vi "WaitForInputData.vi"(0 "Input data timeout":i32=-1 caption="Input data timeout (-1) [ms]" min=-1, 11 "Error in":errorcluster caption="Error in (no error)") -> (4 "Input data timed out?":bool, 6 "Input data names":string[](array[string]), 8 "Input data values":variant[](array[variant]), 15 "Error out":errorcluster)   [LabVIEW 2017, in "VILauncher.lvlib"]
doc: "Waits for <B>Input data names</B> and <B>Input data values</B> sent by a launcher to a dynamic VI using the Run or OpenAndRun function.\n\nThe optional <B>Input data timeout</B> specifies how long time to wait for the input data. Set this to -1 (default) to wait indefinitely. If timeout does occur, <B>Input data timed out?</B> will be True.\n\nThis function does not have to be located in the Top-Level dynamic VI, but can be embedded anywhere in the dynamic VI hierarchy. Just be sure to read the input data before timeout of the Run/OpenAndRun function occurs, or else the input data will be lost.\n\nThis VI is reentrant, and it doesn't run if there is an error on <B>Error in</B>.\n\nSteen Schmidt\nGPower\n30/12 2012"
uses:
  VILauncher.lvlib
panel:
  # "Copyright © 2013\nGPower\nSee enclosed license file for terms and conditions"
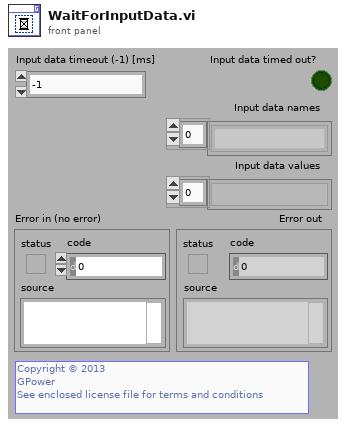
[diagram p1: front panel]
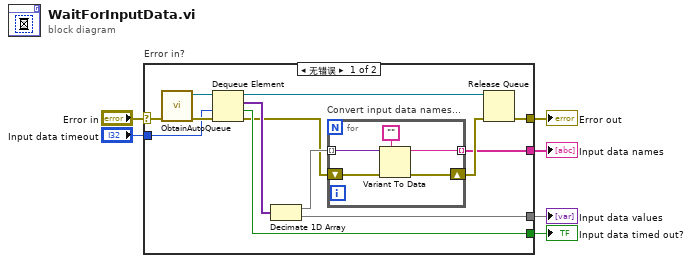
[diagram p0: block diagram]
diagram:
  n1 = case "Error in?" shown="无错误" "Error in" {
    selector: "Error in" -> [w12 w25]
    tunnel: [w16 w25] -> w5
    tunnel: "Input data timeout" -> [w15 _]
    tunnel: [w13 _] -> w3
    tunnel: [w10 _] -> w2
    tunnel: [w7 _] -> w1
    frame No Error {
      n2 = call "ObtainAutoQueue.vi"("Error in"=w12) -> ("Queue"=w18:refnum<queue>, "Error out"=w19:errorcluster)  [unwired: 13 in]
      n3 = Dequeue Element(queue=w18, timeout in ms (-1)=w15, error in (no error)=w19) -> (queue out=w17:refnum<queue>, element=w14:variant[], timed out?=w13:bool, error out=w9:errorcluster)
      n4 = Decimate 1D Array(w14) -> (w11:variant[], w10:variant[])
      n5 = for "Convert input data names..." {
        tunnel: w11 -> [w24] mode=indexing
        shift-right: [w21] -> w8
        shift-left: w9 -> [w22]
        tunnel: [w20] -> w7 mode=indexing
        n6 = Variant To Data(error in=w22, type="", Variant=w24) -> (data=w20:string, error out=w21:errorcluster)
      }
      n7 = Release Queue(queue=w17, error in (no error)=w8) -> (error out=w16:errorcluster)  [unwired: 1 in, 2 out]
    }
    frame Error {
    }
  }
  "Error out" <- w5
  "Input data values" <- w2
  "Input data names" <- w1
  "Input data timed out?" <- w3
